vi "DTtoASCII.vi"(3 "Slide":dbl(slide) scale=0.0..100.0) -> (0 "Numeric":dbl, 1 "ASCII":string)   [LabVIEW 2014]
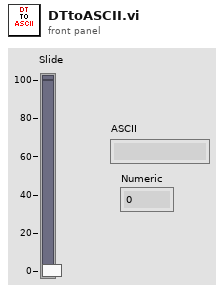
[diagram p1: front panel]
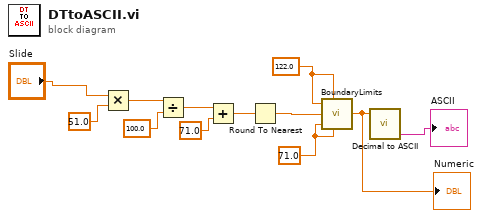
[diagram p0: block diagram]
diagram:
  w8 = 122.0
  w6 = 71.0
  n1 = Multiply(x="Slide", y=51.0) -> (x*y=w12:dbl)
  n2 = Divide(x=w12, y=100.0) -> (x/y=w11:dbl)
  n3 = Add(x=w11, y=71.0) -> (x+y=w10:dbl)
  n4 = Round To Nearest(number=w10) -> (nearest integer value=w7:dbl)
  n5 = call "BoundaryLimits.vi"("UpperLimit"=w8, "UpperValue"=w8, "Input"=w7, "LowerLimit"=w6, "LowerValue"=w6) -> ("Output"=w5:dbl)
  "Numeric" <- w5
  n6 = call "Decimal to ASCII.vi"("Decimal Number"=w5) -> ("ASCII Character"=→"ASCII":string)  [unwired: 2 in, 2 out]
